vi "Virtual Axis Move at Velocity (FW7).vi"(4 "Physical Axis Number (1)":u8=1 min=1, 6 "Relative To (0: virtual axis)":u16(ring) items=["virtual axis", "physical axis"], 7 "Move Speed":i64, 8 "error in (no error)":errorcluster, 9 "Device Number":string, 10 "Virtual Axis Number (1)":u8=1, 11 "VISA resource name":refnum<visa-resource-name>) -> (0 "error out":errorcluster, 3 "VISA resource name out":refnum<visa-resource-name>)   [LabVIEW 2015, in "Zaber A Series.lvlib"]
doc: "Moves a virtual axis at a specified speed. The move speed can be specified for the virtual axis itself or for one of the physical axes comprising it, in which case the other axes will move at proportional speeds.\n\nThe move speed is specified in microstep units for the axis selected. Use the Convert Velocity Units to Device Units VI to convert from standard distance units.\n\nNo responses are returned with this VI, but if you would like to wait until the movement is completed to continue, you can combine this VI with the Poll Until Idle VI. \n\nThis VI requires that the Initialize VI has been called with the same serial port and that the lockstep group has been created with the Lockstep Enable VI."
uses:
  Zaber A Series.lvlib
  Private/All Commands.ctl
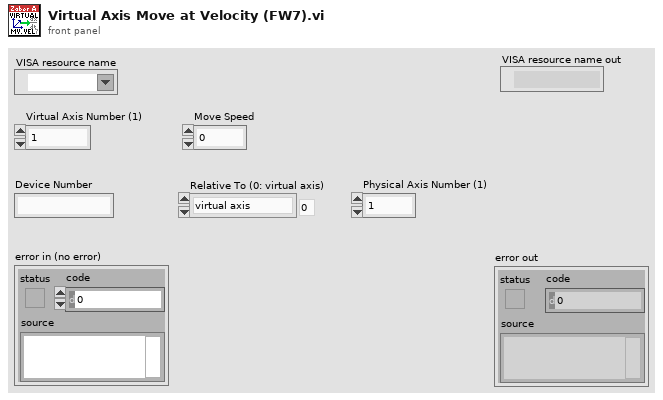
[diagram p1: front panel]
types:
  T1 = typedef "Zaber A Series.lvlib/All Commands.ctl" = string
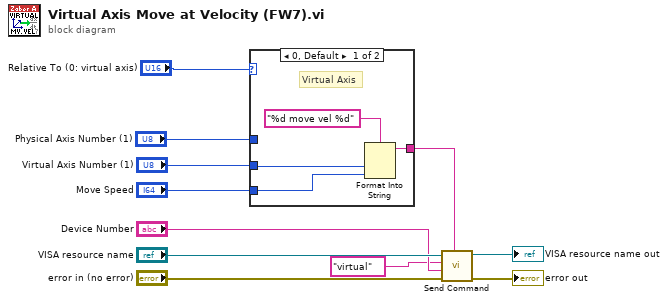
[diagram p0: block diagram]
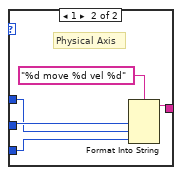
[diagram p2: hidden frame]
diagram:
  n1 = case shown="0, Default" "Relative To (0: virtual axis)" {
    tunnel: [w12 w19] -> w8
    tunnel: "Physical Axis Number (1)" -> [_ w17]
    tunnel: "Virtual Axis Number (1)" -> [w14 w18]
    tunnel: "Move Speed" -> [w13 w16]
    frame 0, Default {
      # "Virtual Axis"
      n2 = Format Into String(format string="%d move vel %d", w14, w13) -> (resulting string=w12:string)  [unwired: 2 in, 1 out]
    }
    frame 1 {
      # "Physical Axis"
      n3 = Format Into String(format string="%d move %d vel %d", w18, w17, w16) -> (resulting string=w19:string)  [unwired: 2 in, 1 out]
    }
  }
  n4 = call "Send Command.vi"("Data"=w8, "error in (no error)"="error in (no error)", "Device and Axis"="Device Number", "Command"=T1 "virtual" ("Complete Command List"), "VISA resource name"="VISA resource name") -> ("error out"=→"error out":errorcluster, "VISA resource name out"=→"VISA resource name out":refnum<visa-resource-name>)  [unwired: 1 in, 4 out]
